vi "Apply.vi"(8 "error in":errorcluster, 11 "HSU MCU V2 in":refnum<class "HSU MCU V2 CFG Simulated.lvclass">) -> (0 "error out":errorcluster, 3 "HSU MCU V2 out":refnum<class "HSU MCU V2 CFG Simulated.lvclass">)   [LabVIEW 2023, in "HSU MCU V2 CFG Simulated.lvclass"]
uses:
  HSU MCU V2 CFG Simulated.lvclass
  Configurations/CFG Base/CFG Base.lvclass/CFG Base.ctl
  HSU MCU V2 CFG/HSU MCU V2 CFG.lvclass
  Configurations/CFG Base/CFG Base.lvclass
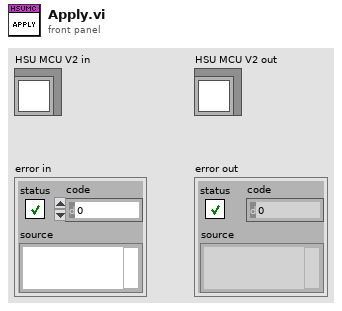
[diagram p1: front panel]
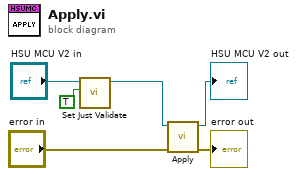
[diagram p0: block diagram]
diagram:
  n1 = call "Set Just Validate.vi"("Just Validate"=TRUE, "CFG Base in"="HSU MCU V2 in") -> ("CFG Base out"=w2:refnum<class "HSU MCU V2 CFG Simulated.lvclass">)  [unwired: 9 in]
  n2 = call-parent "Apply.vi"("error in"="error in", "HSU MCU V2 in"=w2) -> ("error out"=→"error out":errorcluster, "HSU MCU V2 out"=→"HSU MCU V2 out":refnum<class "HSU MCU V2 CFG Simulated.lvclass">)  [unwired: 8 in]
